vi "main.vi"() -> ()   [LabVIEW 2024]
uses:
  typeDef/dataCluster.ctl
  <vilib>/addons/_JKI.lib/REST Client/classes/REST Client/REST Client.lvclass
panel:
  in  "Reset":bool
  out "cos(x)":dbl
  out "sin(x)":dbl
  out "Distance to obstacle":dbl
  out "worldMap":picture
  in  "Base URL":string="http://127.0.0.1:5000"
  out "angle":dbl
  in  "speed":dbl=1.0
  in  "A":bool
  in  "D":bool
  in  "S":bool
  in  "W":bool
  out "Gauge":dbl(knob) scale=0.0..360.0 scale format="%#_12g"
  out "Response body":string
  in  "stop":bool
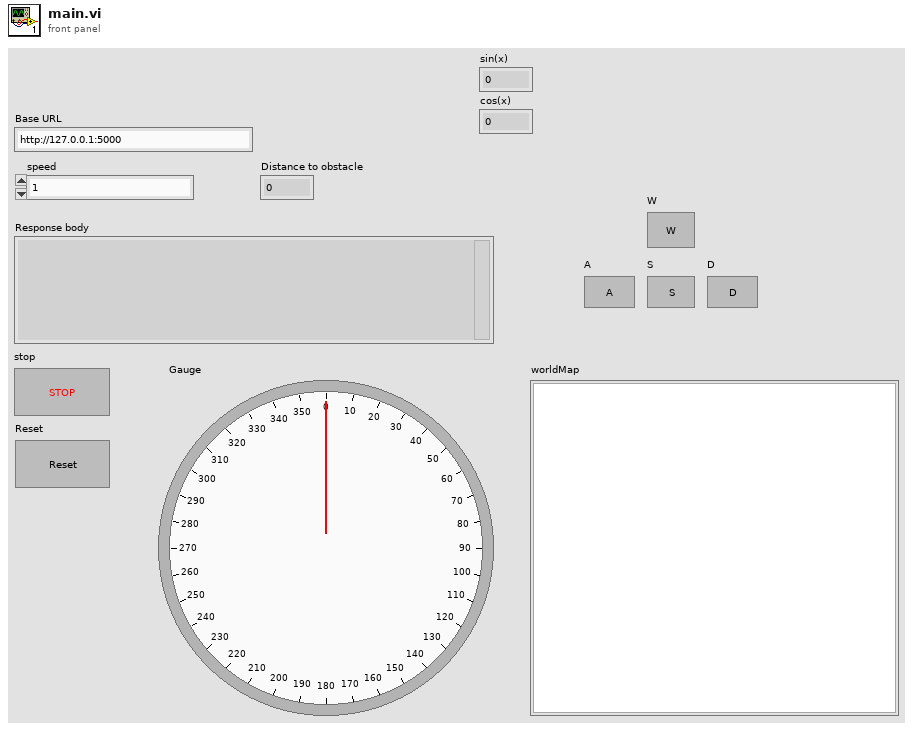
[diagram p1: front panel]
types:
  T1 = cluster{"Width":u16, "Style":enum32{"Solid", "Dash", "Dot", "DashDot", "DashDotDot"}}
  T2 = typedef "dataCluster.ctl" = cluster{"angle":dbl, "turn_left?":bool, "turn_right?":bool, "forward?":bool, "backward?":bool, "stop?":bool, "distance":dbl}
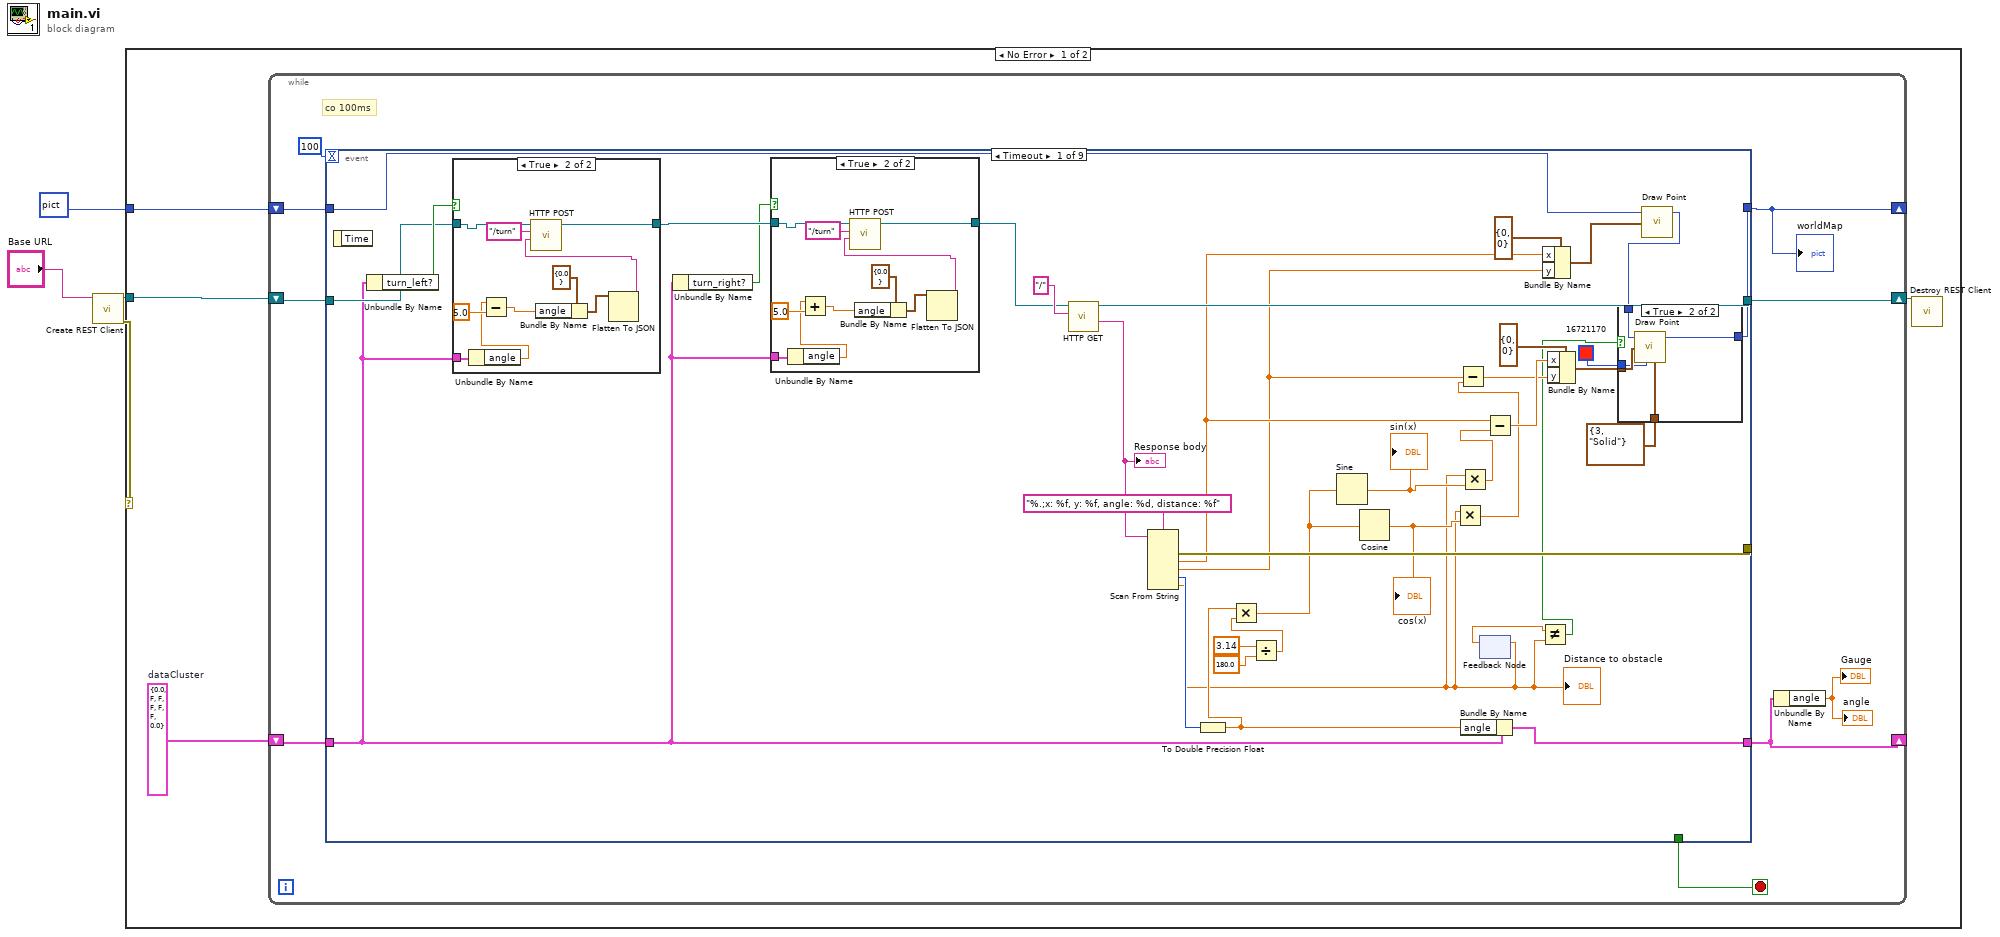
[diagram p0: block diagram]
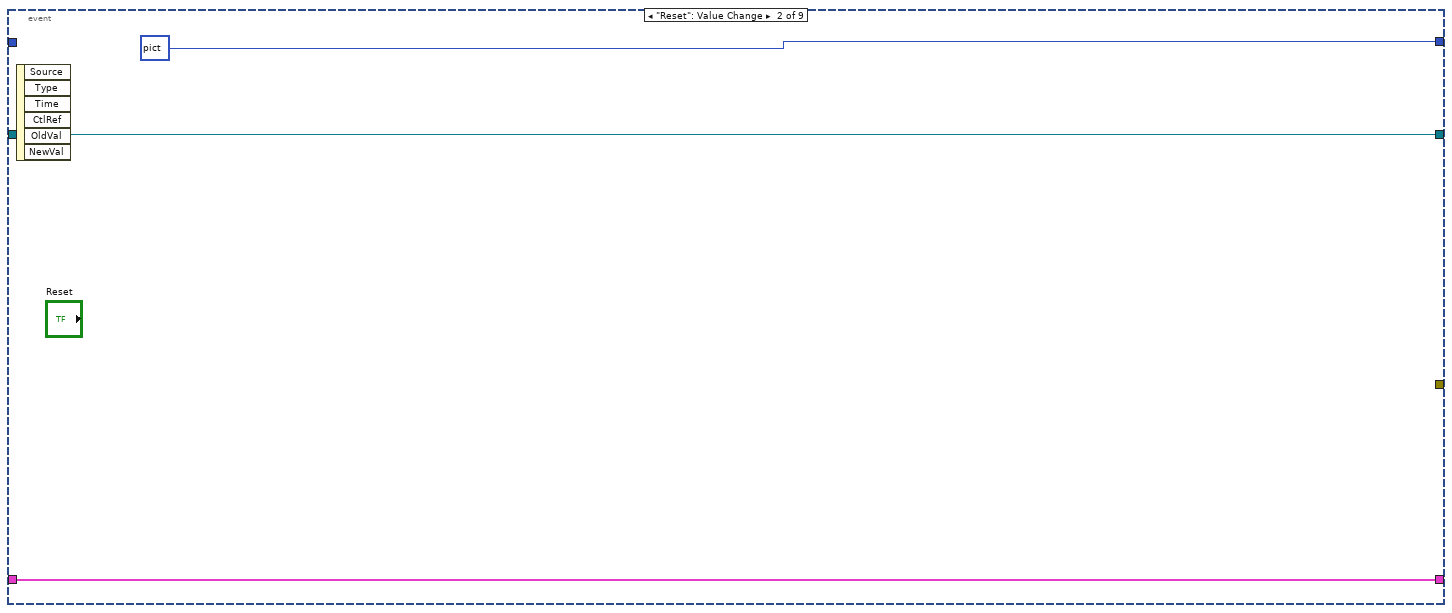
[diagram p5: hidden frame]
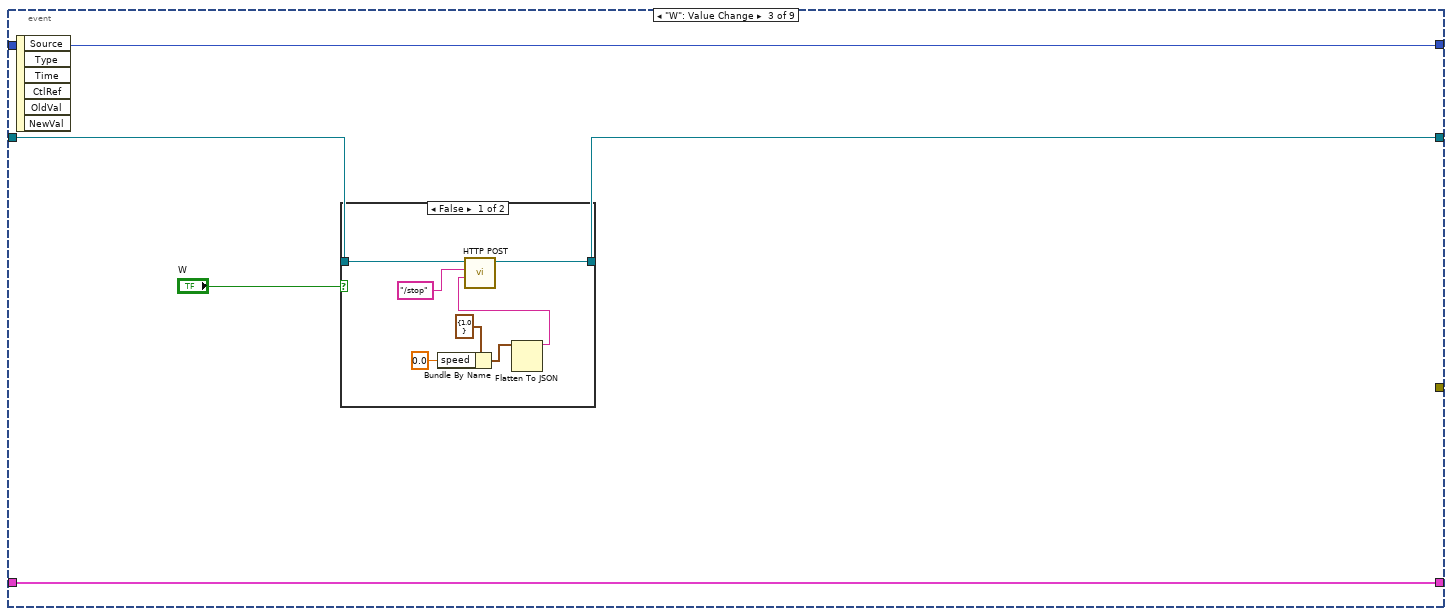
[diagram p6: hidden frame]
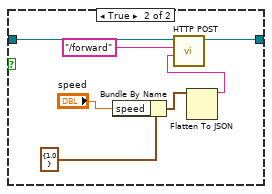
[diagram p7: hidden frame]
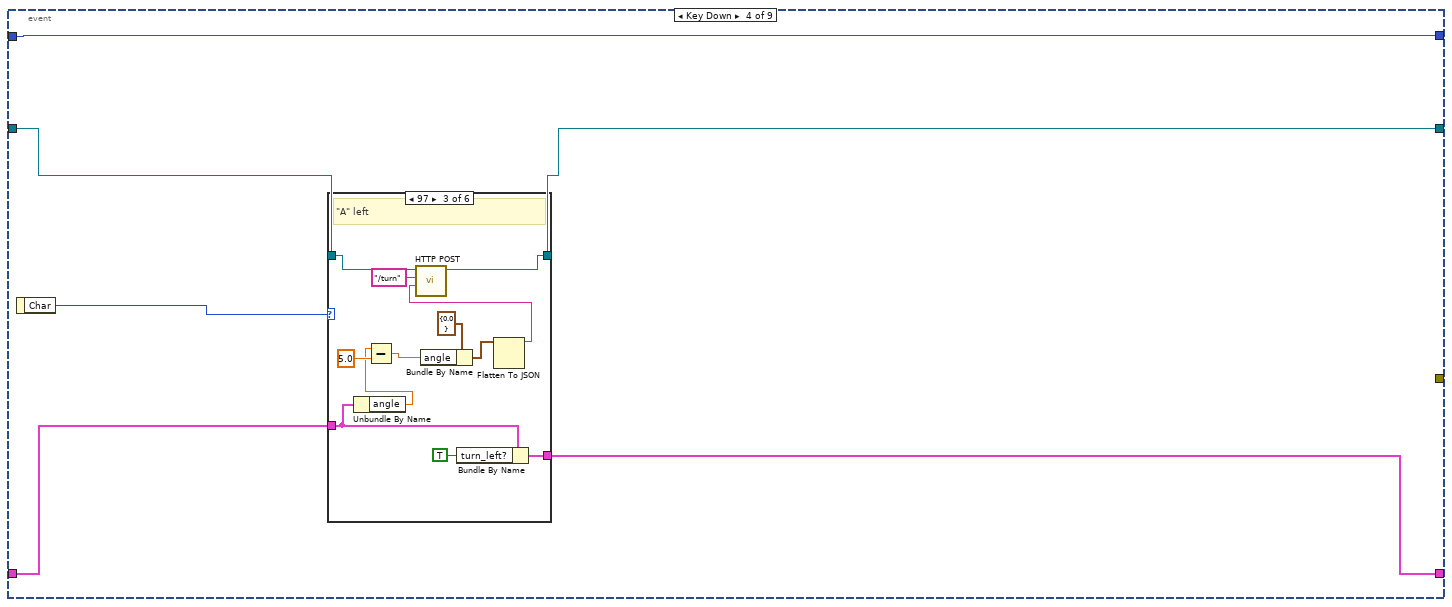
[diagram p8: hidden frame]
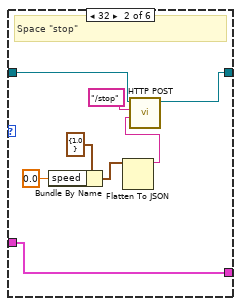
[diagram p10: hidden frame]
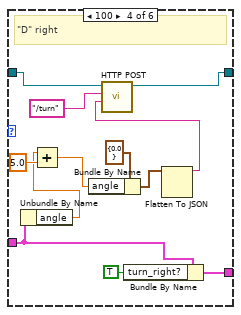
[diagram p11: hidden frame]
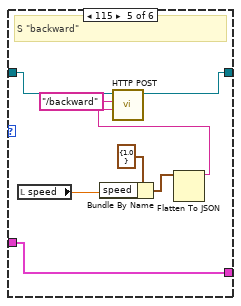
[diagram p12: hidden frame]
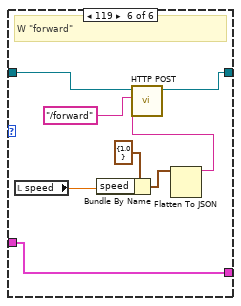
[diagram p13: hidden frame]
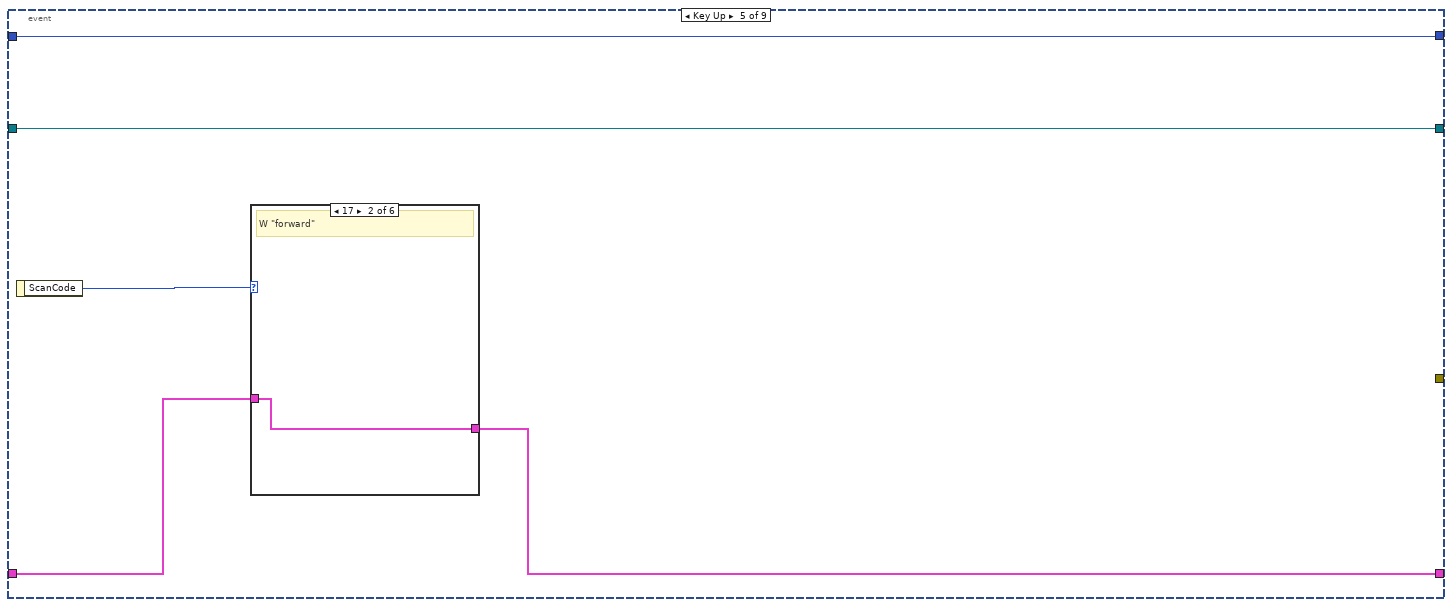
[diagram p14: hidden frame]
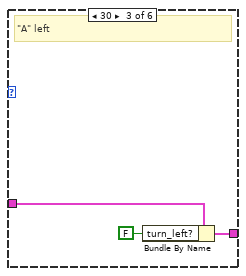
[diagram p16: hidden frame]
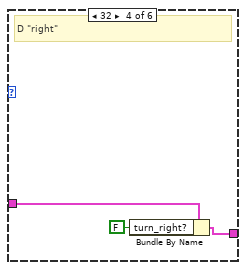
[diagram p17: hidden frame]
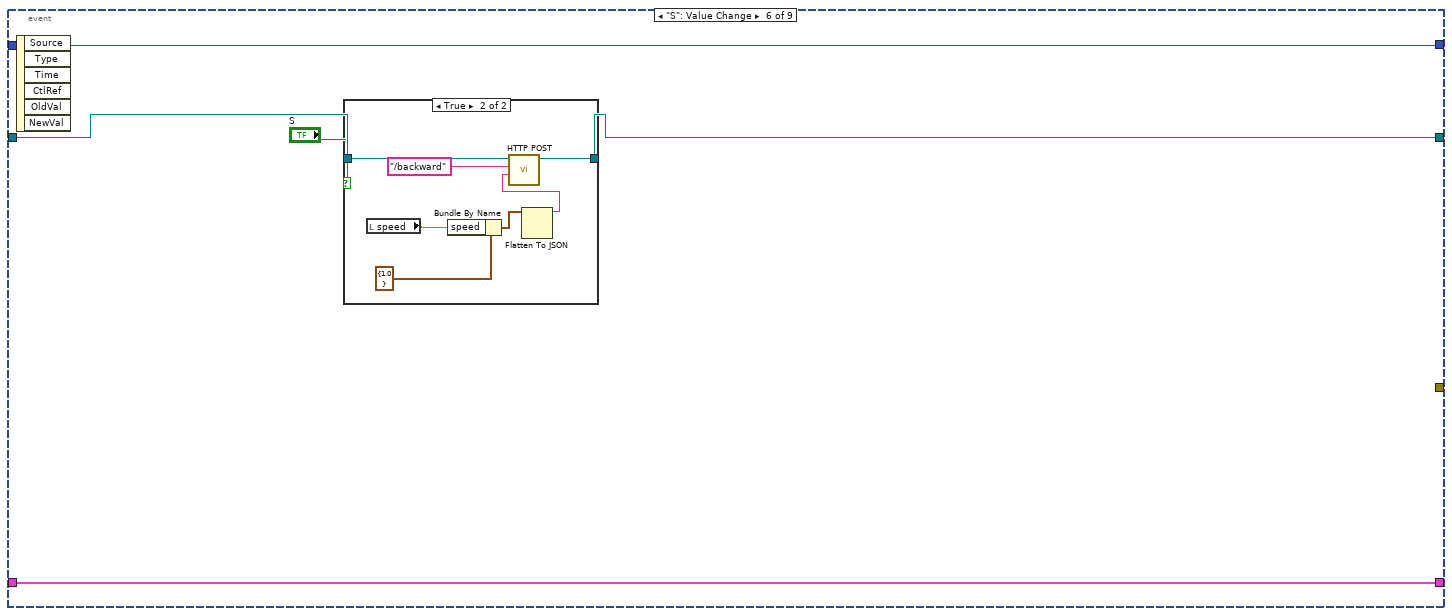
[diagram p20: hidden frame]
diagram:
  n1 = call <vilib>:"Create REST Client.vi"("Base URL"="Base URL") -> ("error out"=w2:errorcluster, "REST Client out"=w3:refnum<class "REST Client.lvclass">)  [unwired: 9 in]
  n2 = case shown="No Error" w2 {
    tunnel: w3 -> [w8 _]
    tunnel: picture data[5B] ("worldMap") -> [w5 _]
    frame No Error {
      w6 = T2 {"angle"=0.0, "turn_left?"=FALSE, "turn_right?"=FALSE, "forward?"=FALSE, "backward?"=FALSE, "stop?"=FALSE, "distance"=0.0}  # dataCluster
      n3 = while {
        shift-right: [w15] -> w7
        shift-left: w8 -> [w14]
        shift-right: [w12] -> _
        shift-left: w6 -> [w13]
        shift-right: [w9] -> _
        shift-left: w5 -> [w10]
        stop <- w17 stop-if-true
        # "co 100ms"
        n4 = event shown="[0] Timeout" {
          selector: _ -> [_ _ _ _ _ _ _ _ _]
          dyn-events: _ -> [_ _ _ _ _ _ _ _ _]
          timeout: 100 -> [_ _ _ _ _ _ _ _ _]
          tunnel: [_ _ _ _ _ _ _ _ "stop"] -> w17
          tunnel: [w55 w86 w90 w107 w166 w180 w200 w222 w242] -> w15
          tunnel: w14 -> [w47 w86 w91 w111 w166 w181 w201 w223 w242]
          tunnel: [w51 _ _ _ _ _ _ _ _] -> _
          tunnel: [w50 w85 w88 w108 w163 w178 w198 w220 w241] -> w12
          tunnel: w13 -> [w44 w85 w88 w109 w164 w178 w198 w220 w241]
          tunnel: w10 -> [w42 _ w87 w106 w162 w177 w196 w218 w240]
          tunnel: [w36 picture data[5B] ("worldMap") w87 w106 w162 w177 w196 w218 w240] -> w9
          event Timeout {
            n5 = event-data() -> ()  [unwired: 1 in, 1 out]
            n6 = Unbundle By Name(w44) -> ("turn_left?"=w48:bool)
            n7 = case shown="True" w48 {
              tunnel: w47 -> [w73 w77]
              tunnel: [w73 w75] -> w46
              tunnel: w44 -> [_ w76]
              frame False {
              }
              frame True {
                n8 = Unbundle By Name(w76) -> ("angle"=w78:dbl)
                n9 = Subtract(x=w78, y=5.0) -> (x-y=w80:dbl)
                n10 = Bundle By Name(cluster=cluster{"angle":dbl} {"angle"=0.0}, "angle"=w80) -> (w82:cluster{"angle":dbl})
                n11 = Flatten To JSON(anything=w82) -> (JSON string=w74:string)  [unwired: 2 in, 1 out]
                n12 = call-dynamic "HTTP POST.vi"("Request body"=w74, "Path"="/turn", "REST Client in"=w77) -> ("REST Client out"=w75:refnum<class "REST Client.lvclass">)  [unwired: 3 in, 5 out]
              }
            }
            n13 = Unbundle By Name(w44) -> ("turn_right?"=w43:bool)
            n14 = case shown="True" w43 {
              tunnel: w46 -> [w62 w66]
              tunnel: [w62 w64] -> w45
              tunnel: w44 -> [_ w65]
              frame False {
              }
              frame True {
                n15 = Unbundle By Name(w65) -> ("angle"=w67:dbl)
                n16 = Add(x=w67, y=5.0) -> (x+y=w69:dbl)
                n17 = Bundle By Name(cluster=cluster{"angle":dbl} {"angle"=0.0}, "angle"=w69) -> (w71:cluster{"angle":dbl})
                n18 = Flatten To JSON(anything=w71) -> (JSON string=w63:string)  [unwired: 2 in, 1 out]
                n19 = call-dynamic "HTTP POST.vi"("Request body"=w63, "Path"="/turn", "REST Client in"=w66) -> ("REST Client out"=w64:refnum<class "REST Client.lvclass">)  [unwired: 3 in, 5 out]
              }
            }
            n20 = call-dynamic "HTTP GET.vi"("Path"="/", "REST Client in"=w45) -> ("Response body"=w53:string, "REST Client out"=w55:refnum<class "REST Client.lvclass">)  [unwired: 4 in, 4 out]
            "Response body" <- w53
            n21 = Scan From String(format string="%.;x: %f, y: %f, angle: %d, distance: %f", input string=w53) -> (error out=w51:errorcluster, output 1=w34:dbl, output 2=w33:dbl, output 3=w49:i32, output 4=w20:dbl)  [unwired: 6 in, 2 out]
            "Distance to obstacle" <- w20
            n22 = To Double Precision Float(number=w49) -> (double precision float=w26:dbl)
            n23 = Divide(x=3.14, y=180.0) -> (x/y=w27:dbl)
            n24 = Multiply(x=w26, y=w27) -> (x*y=w25:dbl)
            n25 = Sine(x=w25) -> (sin(x)=w35:dbl)
            "sin(x)" <- w35
            n26 = Cosine(x=w25) -> (cos(x)=w30:dbl)
            "cos(x)" <- w30
            n27 = Multiply(x=w20, y=w30) -> (x*y=w22:dbl)
            n28 = Subtract(x=w33, y=w22) -> (x-y=w31:dbl)
            n29 = Multiply(x=w20, y=w35) -> (x*y=w21:dbl)
            n30 = Bundle By Name(cluster=w44, "angle"=w26) -> (w50:T2)
            n31 = feedback-in #1(w20) -> ()
            n32 = feedback #1() -> (w19:dbl)  [unwired: 1 in]
            n33 = Subtract(x=w34, y=w21) -> (x-y=w32:dbl)
            n34 = Not Equal?(x=w19, y=w20) -> (x != y?=w18:bool)
            n35 = Bundle By Name(cluster=cluster{"x":i16, "y":i16} {"x"=0, "y"=0} ("point(x,y)"), "x"=w34, "y"=w33) -> (w40:cluster{"x":i16, "y":i16})
            n36 = Bundle By Name(cluster=cluster{"x":i16, "y":i16} {"x"=0, "y"=0} ("point(x,y)"), "x"=w32, "y"=w31) -> (w37:cluster{"x":i16, "y":i16})
            n37 = call <vilib>:"Draw Point.vi"("picture"=w42, "point(x,y)"=w40) -> ("new picture"=w38:picture)  [unwired: 7 in]
            n38 = case shown="True" w18 {
              tunnel: w38 -> [w56 w61]
              tunnel: w37 -> [_ w60]
              tunnel: [w56 w59] -> w36
              tunnel: u32 16721170 ("color(black)") -> [_ w58]
              tunnel: T1 {"Width"=3, "Style"=enum."Solid"} ("pen") -> [_ w57]
              frame False {
              }
              frame True {
                n39 = call <vilib>:"Draw Point.vi"("picture"=w61, "point(x,y)"=w60, "color(black)"=w58, "pen"=w57) -> ("new picture"=w59:picture)  [unwired: 5 in]
              }
            }
          }
          event "Reset": Value Change {
            n40 = event-data() -> ()  [unwired: 1 in, 6 out]
          }
          event "W": Value Change {
            n41 = event-data() -> ()  [unwired: 1 in, 6 out]
            n42 = case shown="False" "W" {
              tunnel: w91 -> [w98 w105]
              tunnel: [w97 w104] -> w90
              frame False {
                n43 = Bundle By Name(cluster=cluster{"speed":dbl} {"speed"=1.0}, "speed"=0.0) -> (w94:cluster{"speed":dbl})
                n44 = Flatten To JSON(anything=w94) -> (JSON string=w92:string)  [unwired: 2 in, 1 out]
                n45 = call-dynamic "HTTP POST.vi"("Request body"=w92, "Path"="/stop", "REST Client in"=w98) -> ("REST Client out"=w97:refnum<class "REST Client.lvclass">)  [unwired: 3 in, 5 out]
              }
              frame True {
                n46 = Bundle By Name(cluster=cluster{"speed":dbl} {"speed"=1.0}, "speed"="speed") -> (w100:cluster{"speed":dbl})
                n47 = Flatten To JSON(anything=w100) -> (JSON string=w99:string)  [unwired: 2 in, 1 out]
                n48 = call-dynamic "HTTP POST.vi"("Request body"=w99, "Path"="/forward", "REST Client in"=w105) -> ("REST Client out"=w104:refnum<class "REST Client.lvclass">)  [unwired: 3 in, 5 out]
              }
            }
          }
          event Key Down {
            n49 = event-data() -> ("Char"=w110:i16)  [unwired: 1 in]
            n50 = case shown="97" w110 {
              tunnel: w111 -> [w113 w120 w130 w143 w150 w161]
              tunnel: [w113 w119 w131 w142 w149 w160] -> w107
              tunnel: w109 -> [w112 w114 w124 w135 w146 w154]
              tunnel: [w112 w114 w122 w134 w146 w154] -> w108
              frame 0, Default {
              }
              frame 32 {
                # "Space \"stop\""
                n51 = Bundle By Name(cluster=cluster{"speed":dbl} {"speed"=1.0}, "speed"=0.0) -> (w117:cluster{"speed":dbl})
                n52 = Flatten To JSON(anything=w117) -> (JSON string=w116:string)  [unwired: 2 in, 1 out]
                n53 = call-dynamic "HTTP POST.vi"("Request body"=w116, "Path"="/stop", "REST Client in"=w120) -> ("REST Client out"=w119:refnum<class "REST Client.lvclass">)  [unwired: 3 in, 5 out]
              }
              frame 97 {
                # "\"A\" left"
                n54 = Unbundle By Name(w124) -> ("angle"=w125:dbl)
                n55 = Subtract(x=w125, y=5.0) -> (x-y=w127:dbl)
                n56 = Bundle By Name(cluster=cluster{"angle":dbl} {"angle"=0.0}, "angle"=w127) -> (w132:cluster{"angle":dbl})
                n57 = Bundle By Name(cluster=w124, "turn_left?"=TRUE) -> (w122:T2)
                n58 = Flatten To JSON(anything=w132) -> (JSON string=w129:string)  [unwired: 2 in, 1 out]
                n59 = call-dynamic "HTTP POST.vi"("Request body"=w129, "Path"="/turn", "REST Client in"=w130) -> ("REST Client out"=w131:refnum<class "REST Client.lvclass">)  [unwired: 3 in, 5 out]
              }
              frame 100 {
                # "\"D\" right"
                n60 = Unbundle By Name(w135) -> ("angle"=w137:dbl)
                n61 = Add(x=w137, y=5.0) -> (x+y=w141:dbl)
                n62 = Bundle By Name(cluster=cluster{"angle":dbl} {"angle"=0.0}, "angle"=w141) -> (w145:cluster{"angle":dbl})
                n63 = Bundle By Name(cluster=w135, "turn_right?"=TRUE ("turn_left?")) -> (w134:T2)
                n64 = Flatten To JSON(anything=w145) -> (JSON string=w139:string)  [unwired: 2 in, 1 out]
                n65 = call-dynamic "HTTP POST.vi"("Request body"=w139, "Path"="/turn" ("Request body"), "REST Client in"=w143) -> ("REST Client out"=w142:refnum<class "REST Client.lvclass">)  [unwired: 3 in, 5 out]
              }
              frame 115 {
                # "S \"backward\""
                n66 = local read "speed"() -> (w152:dbl)
                n67 = Bundle By Name(cluster=cluster{"speed":dbl} {"speed"=1.0}, "speed"=w152) -> (w151:cluster{"speed":dbl})
                n68 = Flatten To JSON(anything=w151) -> (JSON string=w148:string)  [unwired: 2 in, 1 out]
                n69 = call-dynamic "HTTP POST.vi"("Request body"=w148, "Path"="/backward", "REST Client in"=w150) -> ("REST Client out"=w149:refnum<class "REST Client.lvclass">)  [unwired: 3 in, 5 out]
              }
              frame 119 {
                # "W \"forward\""
                n70 = local read "speed"() -> (w157:dbl)
                n71 = Bundle By Name(cluster=cluster{"speed":dbl} {"speed"=1.0}, "speed"=w157) -> (w156:cluster{"speed":dbl})
                n72 = Flatten To JSON(anything=w156) -> (JSON string=w155:string)  [unwired: 2 in, 1 out]
                n73 = call-dynamic "HTTP POST.vi"("Request body"=w155, "Path"="/forward", "REST Client in"=w161) -> ("REST Client out"=w160:refnum<class "REST Client.lvclass">)  [unwired: 3 in, 5 out]
              }
            }
          }
          event Key Up {
            n74 = event-data() -> ("ScanCode"=w165:i16)  [unwired: 1 in]
            n75 = case shown="17" w165 {
              tunnel: w164 -> [w167 w168 w171 w173 w175 w176]
              tunnel: [w167 w168 w169 w172 w175 w176] -> w163
              frame 0, Default {
              }
              frame 17 {
                # "W \"forward\""
              }
              frame 30 {
                # "\"A\" left"
                n76 = Bundle By Name(cluster=w171, "turn_left?"=FALSE) -> (w169:T2)
              }
              frame 32 {
                # "D \"right\""
                n77 = Bundle By Name(cluster=w173, "turn_right?"=FALSE ("turn_left?")) -> (w172:T2)
              }
              frame 31 {
                # "S \"backward\""
              }
              frame 57 {
                # "Space \"stop\""
              }
            }
          }
          event "S": Value Change {
            n78 = event-data() -> ()  [unwired: 1 in, 6 out]
            n79 = case shown="True" "S" {
              tunnel: w181 -> [w188 w195]
              tunnel: [w187 w194] -> w180
              frame False {
                n80 = Bundle By Name(cluster=cluster{"speed":dbl} {"speed"=1.0}, "speed"=0.0) -> (w184:cluster{"speed":dbl})
                n81 = Flatten To JSON(anything=w184) -> (JSON string=w182:string)  [unwired: 2 in, 1 out]
                n82 = call-dynamic "HTTP POST.vi"("Request body"=w182, "Path"="/stop", "REST Client in"=w188) -> ("REST Client out"=w187:refnum<class "REST Client.lvclass">)  [unwired: 3 in, 5 out]
              }
              frame True {
                n83 = local read "speed"() -> (w189:dbl)
                n84 = Bundle By Name(cluster=cluster{"speed":dbl} {"speed"=1.0}, "speed"=w189) -> (w191:cluster{"speed":dbl})
                n85 = Flatten To JSON(anything=w191) -> (JSON string=w190:string)  [unwired: 2 in, 1 out]
                n86 = call-dynamic "HTTP POST.vi"("Request body"=w190, "Path"="/backward", "REST Client in"=w195) -> ("REST Client out"=w194:refnum<class "REST Client.lvclass">)  [unwired: 3 in, 5 out]
              }
            }
          }
          event "D": Value Change {
            n87 = event-data() -> ()  [unwired: 1 in, 6 out]
            n88 = Unbundle By Name(w198) -> ("angle"=w197:dbl)
            n89 = case shown="False" "D" {
              tunnel: w201 -> [w208 w217]
              tunnel: [w207 w216] -> w200
              tunnel: w197 -> [w203 w210]
              frame False {
                n90 = Bundle By Name(cluster=cluster{"angle":dbl} {"angle"=1.0}, "angle"=w203) -> (w204:cluster{"angle":dbl})
                n91 = Flatten To JSON(anything=w204) -> (JSON string=w202:string)  [unwired: 2 in, 1 out]
                n92 = call-dynamic "HTTP POST.vi"("Request body"=w202, "Path"="/right", "REST Client in"=w208) -> ("REST Client out"=w207:refnum<class "REST Client.lvclass">)  [unwired: 3 in, 5 out]
              }
              frame True {
                n93 = Add(x=w210, y=5.0) -> (x+y=w211:dbl)
                n94 = Bundle By Name(cluster=cluster{"angle":dbl} {"angle"=1.0}, "angle"=w211) -> (w213:cluster{"angle":dbl})
                n95 = Flatten To JSON(anything=w213) -> (JSON string=w212:string)  [unwired: 2 in, 1 out]
                n96 = call-dynamic "HTTP POST.vi"("Request body"=w212, "Path"="/turn", "REST Client in"=w217) -> ("REST Client out"=w216:refnum<class "REST Client.lvclass">)  [unwired: 3 in, 5 out]
              }
            }
          }
          event "A": Value Change {
            n97 = event-data() -> ()  [unwired: 1 in, 6 out]
            n98 = Unbundle By Name(w220) -> ("angle"=w219:dbl)
            n99 = case shown="True" "A" {
              tunnel: w223 -> [w230 w239]
              tunnel: [w229 w238] -> w222
              tunnel: w219 -> [w225 w232]
              frame False {
                n100 = Bundle By Name(cluster=cluster{"angle":dbl} {"angle"=1.0}, "angle"=w225) -> (w226:cluster{"angle":dbl})
                n101 = Flatten To JSON(anything=w226) -> (JSON string=w224:string)  [unwired: 2 in, 1 out]
                n102 = call-dynamic "HTTP POST.vi"("Request body"=w224, "Path"="/turn", "REST Client in"=w230) -> ("REST Client out"=w229:refnum<class "REST Client.lvclass">)  [unwired: 3 in, 5 out]
              }
              frame True {
                n103 = Subtract(x=w232, y=5.0) -> (x-y=w233:dbl)
                n104 = Bundle By Name(cluster=cluster{"angle":dbl} {"angle"=1.0}, "angle"=w233) -> (w235:cluster{"angle":dbl})
                n105 = Flatten To JSON(anything=w235) -> (JSON string=w234:string)  [unwired: 2 in, 1 out]
                n106 = call-dynamic "HTTP POST.vi"("Request body"=w234, "Path"="/left", "REST Client in"=w239) -> ("REST Client out"=w238:refnum<class "REST Client.lvclass">)  [unwired: 3 in, 5 out]
              }
            }
          }
          event "stop": Value Change {
            n107 = event-data() -> ()  [unwired: 1 in, 6 out]
          }
        }
        "worldMap" <- w9
        n108 = Unbundle By Name(w12) -> ("angle"=→"angle" →"Gauge":dbl)
      }
      n109 = call-dynamic "Destroy REST Client.vi"("REST Client in"=w7) -> ()  [unwired: 10 in, 1 out]
    }
    frame Error {
      n110 = One Button Dialog(message="Problem with host") -> ()  [unwired: 1 in, 1 out]
    }
  }
